vi "Console_Reconnect.vi"(11 "Queue in":refnum<queue>) -> ()   [LabVIEW 2022 SP3]
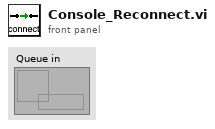
[diagram p1: front panel]
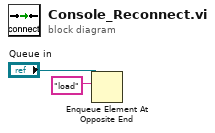
[diagram p0: block diagram]
diagram:
  n1 = Enqueue Element At Opposite End(queue="Queue in", element="load") -> ()  [unwired: 2 in, 3 out]
